vi "MicrophoneColdSpray_Complete_Descriptors_v10.vi"() -> ()   [LabVIEW 2015]
uses:
  <vilib>/Analysis/4window.llb/Hanning Window (DBL).vi
  <vilib>/Analysis/4window.llb/Hamming Window (DBL).vi
  <vilib>/Analysis/4window.llb/Blackman-Harris Window (DBL).vi
  <vilib>/Analysis/4window.llb/Exact Blackman Window (DBL).vi
  <vilib>/Analysis/4window.llb/Blackman Window (DBL).vi
  <vilib>/Analysis/4window.llb/Flat Top Window (DBL).vi
  <vilib>/Analysis/4window.llb/Blackman-Nuttall Window (DBL).vi
  <vilib>/Analysis/4window.llb/Triangle Window (DBL).vi
  <vilib>/Analysis/4window.llb/Modified Bartlett-Hanning Window (DBL).vi
  <vilib>/Analysis/4window.llb/Bohman Window (DBL).vi
  <vilib>/Analysis/4window.llb/Parzen Window (DBL).vi
  <vilib>/Analysis/4window.llb/Welch Window (DBL).vi
  <vilib>/Analysis/4window.llb/AllCosWindow (DBL).vi
  <vilib>/Analysis/0measdsp.llb/Scaled Time Domain Window (DBL).vi
  <vilib>/Analysis/NI_AALPro.lvlib
panel:
  in  "Window Type":u16(ring) items=["Rectangle", "Hanning", "Hamming", "Blackman-Harris", "Exact Blackman", "Blackman", "Flat Top", "Empty1", "Empty2", "Empty3", "Empty4", "Blackman Nuttall", "Empty5", "Empty6", "Empty7", "Empty8", "Empty9", "Empty10", "Empty11", "Empty12", "Empty13", "Empty14", "Empty15", "Empty16", "Empty17", "Empty18", "Empty19", "Empty20", "Empty21", "Empty22", "Triangle", "Bartlett-Hanning", "Bohman", "Parzen", "Welch"]
  out "Boolean 3":bool=TRUE
  out "Boolean 2":bool=TRUE
  out "Boolean":bool=TRUE
  out "DPC":string
  out "Queue Status Check":string
  out "DAC":string
  out "Number of Elements in Queue":i32(knob) scale=0.0..15.0
  out "Microphone Sensitivity":i32=450
  in  "Path to Save Folder for Collected Sound Data":path=path "H:/LabVIEW 2015 Projects/ColdSprayMic/TestDev"
  out "Signal 1":bool
  out "Signal 3":bool
  out "Signal 2":bool
  in  "Noise Amplitude (V) 3":dbl=0.01
  in  "Amplitude (V) 3":dbl=0.3
  in  "Frequency (Hz) 3":dbl=5000.0
  in  "Noise Amplitude (V) 2":dbl=0.02
  in  "Amplitude (V) 2":dbl=0.5
  in  "Frequency (Hz) 2":dbl=2000.0
  in  "Noise Amplitude (V)":dbl=0.3
  in  "Amplitude (V)":dbl=1.0
  in  "Frequency (Hz)":dbl=500.0
  in  "Real Data?":u16(ring) items=["Yes", "No"]
  out "Baseline Spectral Centroid":dbl
  out "Baseline Spectral Spread":dbl
  out "Spectal Descriptors":cluster{dbl, dbl, "t":dbl, dbl}(graph)
  out "Rolling STFT":dbl[][](graph)
  in  "Device Name":tag="cDAQ1Mod1"
  in  "Rate (Hz)":dbl=51200.0
  in  "Number of Samples per Read":i32=4096
  in  "Rolling Buffer (s) MAX 20s":dbl=4.0
  out "Start Time and Date":timestamp
  in  "File Name for Collected Sound Data":string="TestName"
  out "Live Audio":dynamicdata(graph) caption="Waveform Chart"
  in  "stop (F)":bool caption="Stop"
  # "Settings"
  # "Live Signal and Processing"
  # "Real Data = Yes"
  # "Real Data = No"
  # "Simulated Signals"
  # "- Settings for Simulated Signal\n- 10 secs of Signal 1, 10s of Signal 1+2, 10s of Signal 1+2+3, 10s of Signal 1+2, and repeat\n- Set \"Number of Samples per Read\" to 4096 to test with Simulated Signals"
  # "Simulated Signal 1 - Baseline - Sine with Inverse F Noise"
  # "Current Signals"
  # "Program Status"
  # "Simulated Signal 2 - Sine with Inverse F Noise"
  # "Simulated Signal 3  - Sine with Inverse F Noise"
  # "For All Testing"
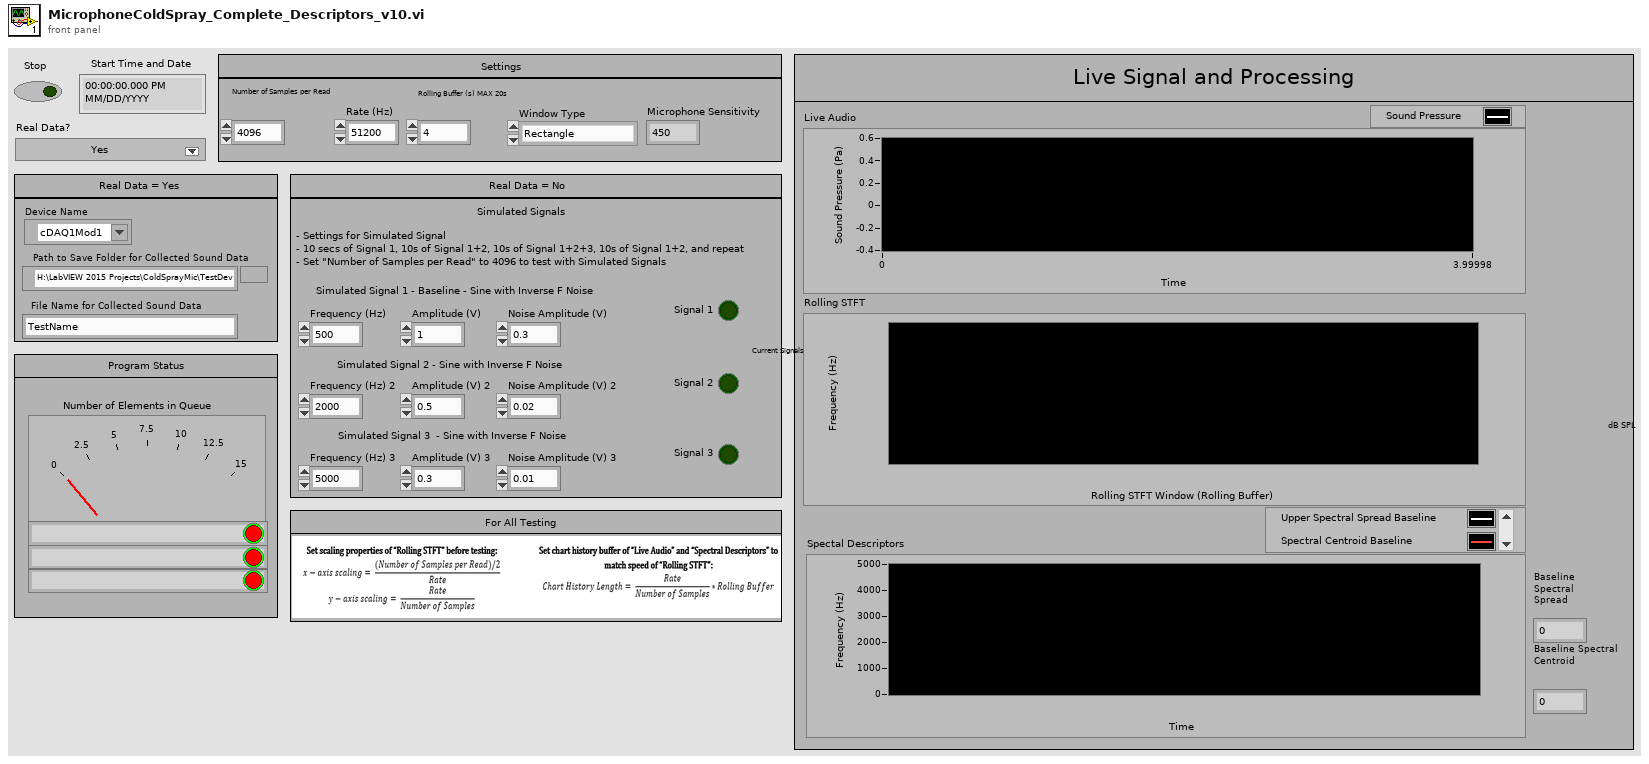
[diagram p1: front panel]
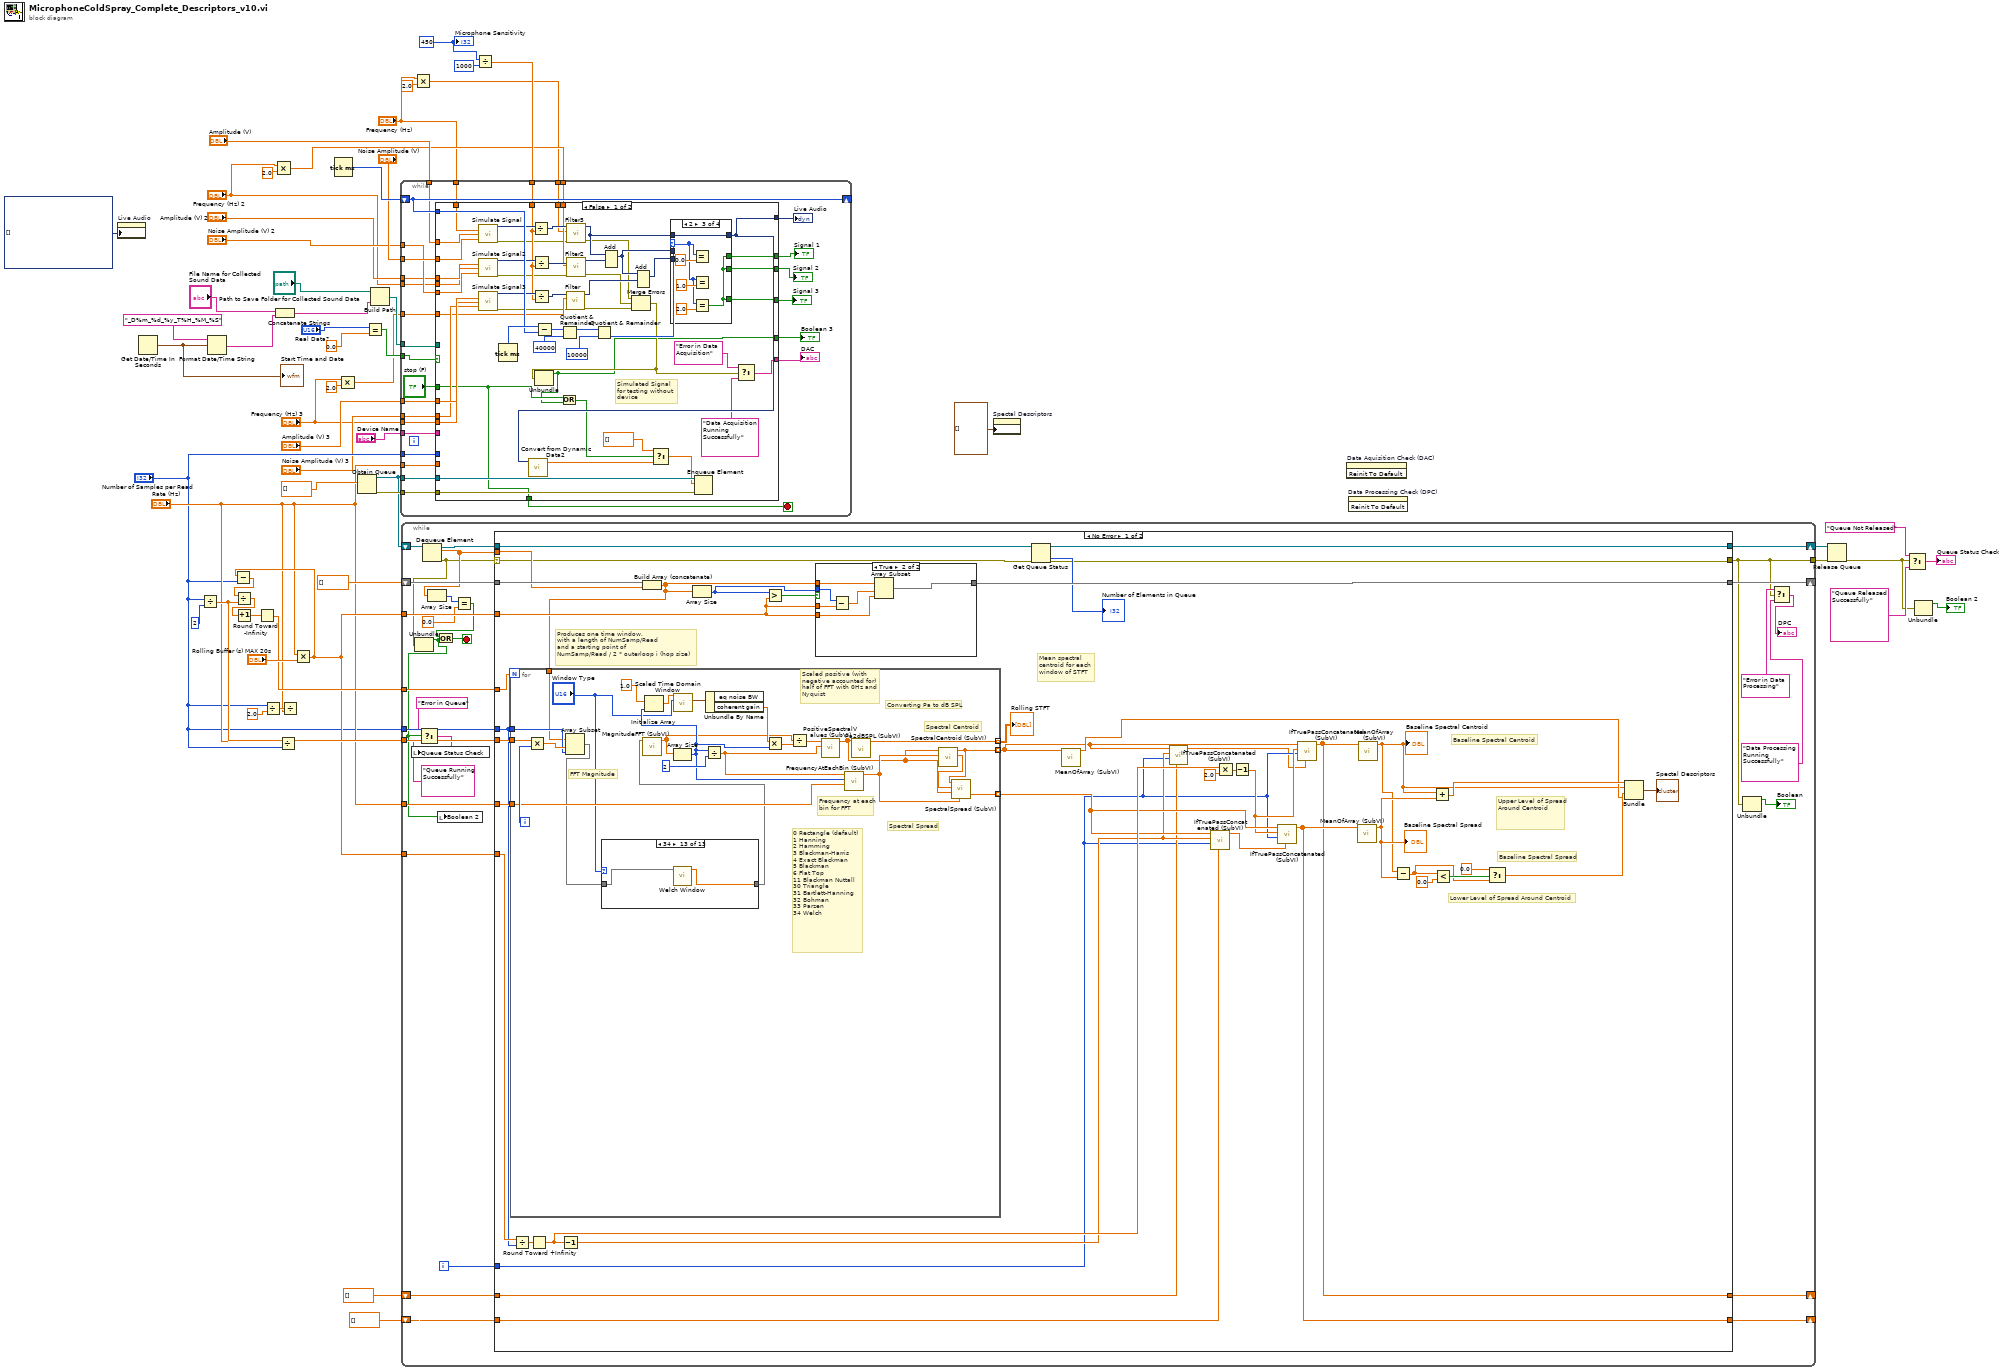
[diagram p0: block diagram]
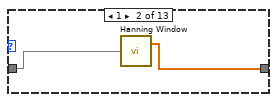
[diagram p4: hidden frame]
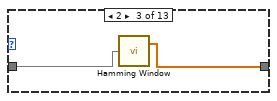
[diagram p5: hidden frame]
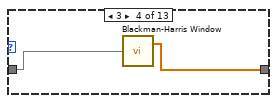
[diagram p6: hidden frame]
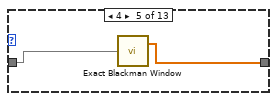
[diagram p7: hidden frame]
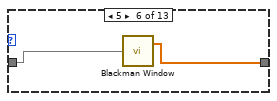
[diagram p8: hidden frame]
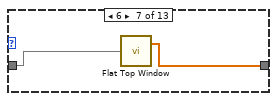
[diagram p9: hidden frame]
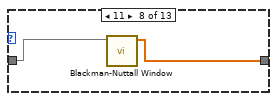
[diagram p10: hidden frame]
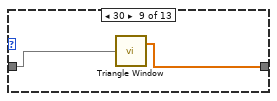
[diagram p11: hidden frame]
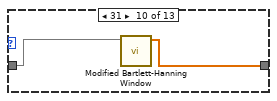
[diagram p12: hidden frame]
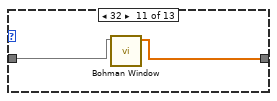
[diagram p13: hidden frame]
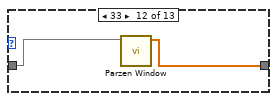
[diagram p14: hidden frame]
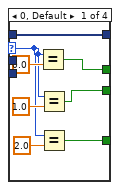
[diagram p16: hidden frame]
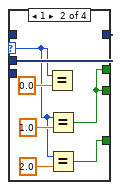
[diagram p17: hidden frame]
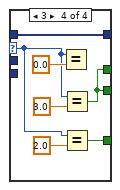
[diagram p18: hidden frame]
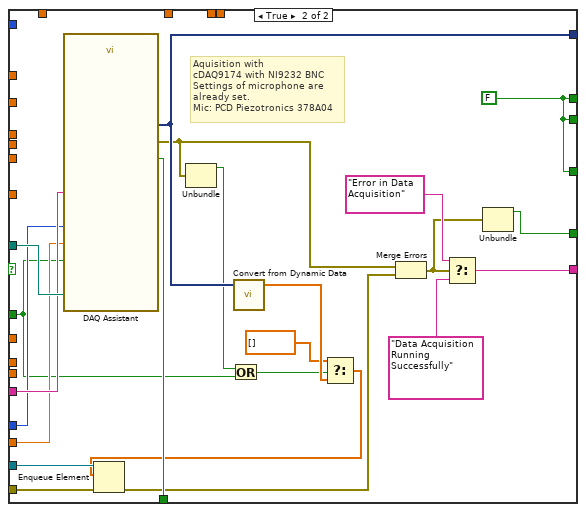
[diagram p19: hidden frame]
diagram:
  w22 = 450
  n1 = property on="Live Audio" class="WFChart (strict)"("History Data"=dynamicdata[] []) -> ()  [unwired: 2 in, 2 out]
  n2 = Get Date/Time In Seconds() -> (seconds since 1Jan1904=w53:timestamp)
  "Start Time and Date" <- w53
  n3 = Divide(x="Number of Samples per Read", y=2) -> (x/y=w45:dbl)
  n4 = Format Date/Time String(time format string (%c)="_D%m_%d_%y_T%H_%M_%S", seconds (now)=w53) -> (date/time string=w55:string)  [unwired: 1 in]
  n5 = Divide(x="Number of Samples per Read", y=2.0) -> (x/y=w38:dbl)
  n6 = Multiply(x="Frequency (Hz) 2", y=2.0) -> (x*y=w15:dbl)
  n7 = Concatenate Strings("File Name for Collected Sound Data", w55) -> (w54:string)
  n8 = Divide(x="Rate (Hz)", y="Number of Samples per Read") -> ()  [unwired: 1 out]
  n9 = Divide(x=w38, y="Rate (Hz)") -> ()  [unwired: 1 out]
  n10 = Multiply(x="Rate (Hz)", y="Rolling Buffer (s) MAX 20s") -> (x*y=w40:dbl)
  n11 = Subtract(x=w40, y="Number of Samples per Read") -> (x-y=w47:dbl)
  n12 = Divide(x=w47, y=w45) -> (x/y=w50:dbl)
  n13 = Increment(x=w50) -> (x+1=w49:dbl)
  n14 = Round Toward -Infinity(1:w49) -> (0:w44:dbl)
  n15 = Tick Count (ms)() -> (millisecond timer value=w31:u32)
  n16 = Multiply(x="Frequency (Hz) 3", y=2.0) -> (x*y=w19:dbl)
  n17 = Obtain Queue(element data type=dbl[] []) -> (queue out=w9:refnum<queue>, error out=w10:errorcluster)  [unwired: 4 in, 1 out]
  n18 = Equal?(x="Real Data?", y=0.0) -> (x = y?=w32:bool)
  n19 = Build Path(base path="Path to Save Folder for Collected Sound Data", name or relative path=w54) -> (appended path=w52:path)
  n20 = while {
    tunnel: w45 -> [w88]
    tunnel: w44 -> [w87]
    tunnel: "Number of Samples per Read" -> [w75]
    tunnel: w40 -> [w86]
    shift-right: [w82] -> _
    shift-left: dbl[] [] -> [w85]
    shift-right: [w83] -> _
    shift-left: dbl[] [] -> [w84]
    tunnel: w40 -> [w81]
    shift-right: [w80] -> w7
    shift-left: w9 -> [w74]
    shift-right: [w79] -> _
    shift-left: dbl[] [] -> [w76]
    tunnel: "Rate (Hz)" -> [w78]
    tunnel: [w59] -> w6
    i -> [w77]
    stop <- w71 stop-if-true
    n21 = Dequeue Element(queue=w74) -> (queue out=w73:refnum<queue>, element=w68:dbl[], error out=w61:errorcluster)  [unwired: 2 in, 1 out]
    n22 = Unbundle(w61) -> ("status"=w58:bool)  [unwired: 2 out]
    n23 = Select(t="Error in Queue", s=w58, f="Queue Running Successfully") -> (s? t:f=w62:string)
    n24 = local write "Queue Status Check"(w62) -> ()
    n25 = Array Size(array=w68) -> (size(s)=w69:i32)
    n26 = local write "Boolean 2"(w58) -> ()
    n27 = Equal?(x=w69, y=0.0) -> (x = y?=w72:bool)
    n28 = Or(x=w72, y=w58) -> (x .or. y?=w71:bool)
    n29 = case shown="No Error" w61 {
      selector: w61 -> [w89 w189]
      tunnel: w88 -> [w118 _]
      tunnel: w87 -> [w117 _]
      tunnel: w86 -> [w116 _]
      tunnel: w85 -> [w99 w193]
      tunnel: w84 -> [w115 w192]
      tunnel: [w103 w192] -> w83
      tunnel: [w94 w193] -> w82
      tunnel: w81 -> [w112 _]
      tunnel: [w92 w190] -> w80
      tunnel: [w111 w191] -> w79
      tunnel: w78 -> [w110 _]
      tunnel: w77 -> [w97 _]
      tunnel: w76 -> [w108 w191]
      tunnel: w75 -> [w107 _]
      tunnel: w73 -> [w93 w190]
      tunnel: w68 -> [w106 _]
      tunnel: [w90 w189] -> w59
      frame No Error {
        # "Produces one time window,\nwith a length of NumSamp/Read\nand a starting point of \nNumSamp/Read / 2 * outerloop i (hop size)"
        # "Mean spectral centroid for each window of STFT"
        # "Upper Level of Spread Around Centroid"
        # "Lower Level of Spread Around Centroid"
        # "Baseline Spectral Centroid"
        # "Baseline Spectral Spread"
        n30 = Divide(x=w116, y=w107) -> (x/y=w130:dbl)
        n31 = Round Toward +Infinity(x=w130) -> (ceil(x): smallest int >= x=w127:dbl)
        n32 = Decrement(x=w127) -> (x-1=w100:dbl)
        n33 = Build Array (concatenate)(w108, w106) -> (w109:dbl[])
        n34 = for {
          N: w117 -> [_]
          tunnel: [w161] -> w131 mode=indexing
          tunnel: [w159] -> w96 mode=indexing
          tunnel: [w156] -> w104 mode=indexing
          tunnel: w118 -> [w154]
          tunnel: w107 -> [w153]
          tunnel: w110 -> [w152]
          tunnel: w109 -> [w151]
          i -> [w160]
          # "0 Rectangle (default) \n1 Hanning \n2 Hamming \n3 Blackman-Harris \n4 Exact Blackman \n5 Blackman \n6 Flat Top \n11 Blackman Nuttall \n30 Triangle \n31 Bartlett-Hanning \n32 Bohman \n33 Parzen \n34 Welch"
          # "FFT Magnitude"
          # "Converting Pa to dB SPL"
          # "Scaled positive (with negative accounted for) half of FFT with 0Hz and Nyquist"
          # "Frequency at each bin for FFT"
          # "Spectral Spread"
          # "Spectral Centroid"
          n35 = Multiply(x=w154, y=w160) -> (x*y=w163:dbl)
          n36 = Array Subset(array=w151, index=w163, length=w153) -> (w141:dbl[])
          n37 = case shown="34" "Window Type" {
            tunnel: w141 -> [w164 w166 w168 w170 w172 w174 w176 w178 w180 w182 w184 w186 w188]
            tunnel: [w164 w165 w167 w169 w171 w173 w175 w177 w179 w181 w183 w185 w187] -> w140
            frame 0, Default {
            }
            frame 1 {
              n38 = call-poly <vilib>:"Hanning Window.vi"("X"=w166) -> ("Windowed X"=w165:dbl[])  [unwired: 1 out]
            }
            frame 2 {
              n39 = call-poly <vilib>:"Hamming Window.vi"("X"=w168) -> ("Windowed X"=w167:dbl[])  [unwired: 1 out]
            }
            frame 3 {
              n40 = call-poly <vilib>:"Blackman-Harris Window.vi"("X"=w170) -> ("Windowed X"=w169:dbl[])  [unwired: 1 out]
            }
            frame 4 {
              n41 = call-poly <vilib>:"Exact Blackman Window.vi"("X"=w172) -> ("Windowed X"=w171:dbl[])  [unwired: 1 out]
            }
            frame 5 {
              n42 = call-poly <vilib>:"Blackman Window.vi"("X"=w174) -> ("Windowed X"=w173:dbl[])  [unwired: 1 out]
            }
            frame 6 {
              n43 = call-poly <vilib>:"Flat Top Window.vi"("X"=w176) -> ("Windowed X"=w175:dbl[])  [unwired: 1 out]
            }
            frame 11 {
              n44 = call-poly <vilib>:"Blackman-Nuttall Window.vi"("X"=w178) -> ("Windowed X"=w177:dbl[])  [unwired: 9 in, 1 out]
            }
            frame 30 {
              n45 = call-poly <vilib>:"Triangle Window.vi"("X"=w180) -> ("Windowed X"=w179:dbl[])  [unwired: 1 out]
            }
            frame 31 {
              n46 = call-poly <vilib>:"Modified Bartlett-Hanning Window.vi"("X"=w182) -> ("Windowed X"=w181:dbl[])  [unwired: 9 in, 1 out]
            }
            frame 32 {
              n47 = call-poly <vilib>:"Bohman Window.vi"("X"=w184) -> ("Windowed X"=w183:dbl[])  [unwired: 9 in, 1 out]
            }
            frame 33 {
              n48 = call-poly <vilib>:"Parzen Window.vi"("X"=w186) -> ("Windowed X"=w185:dbl[])  [unwired: 9 in, 1 out]
            }
            frame 34 {
              n49 = call-poly <vilib>:"Welch Window.vi"("X"=w188) -> ("Windowed X"=w187:dbl[])  [unwired: 9 in, 1 out]
            }
          }
          n50 = call "MagnitudeFFT (SubVI).vi"("Windowed Signal Array"=w140) -> ("Magnitude FFT"=w143:dbl[])  [unwired: 10 in]
          n51 = Array Size(array=w143) -> (size(s)=w144:i32)
          n52 = Initialize Array(1.0 ("element"), w144) -> (w145:dbl[])
          n53 = call-poly <vilib>:"Scaled Time Domain Window.vi"("window"="Window Type", "X"=w145) -> ("window properties"=w148:cluster{"eq noise BW":dbl, "coherent gain":dbl})  [unwired: 1 in, 8 out]
          n54 = Unbundle By Name(w148) -> ("coherent gain"=w147:dbl)  [unwired: 1 out]
          n55 = Divide(x=w144, y=2) -> (x/y=w155:dbl)
          n56 = Multiply(x=w147, y=w144) -> (x*y=w146:dbl)
          n57 = Divide(x=w143, y=w146) -> (x/y=w142:dbl[])
          n58 = call "PositiveSpectralValues (SubVI).vi"("Size of Positive Half of FFT"=w155, "Scaled Full Length FFT"=w142) -> ("Positve Half of FFT with 0Hz and Nyquist"=w150:dbl[])  [unwired: 9 in]
          n59 = call "FrequencyAtEachBin (SubVI).vi"("Rate of Measurement (Hz)"=w152, "Length of Full FFT"=w144, "Length of Positive Half of FFT"=w155) -> ("Frequency Array"=w158:dbl[])  [unwired: 8 in]
          n60 = call "Pa2dBSPL (SubVI).vi"("Positve Half of FFT with 0Hz and Nyquist"=w150) -> ("dB SPL"=w161:dbl[])  [unwired: 10 in]
          n61 = call "SpectralCentroid (SubVI).vi"("Frequency Array"=w158, "Positve Half of FFT with 0Hz and Nyquist"=w150) -> ("Sum of FFT Mags"=w157:dbl, "Spectral Centroid"=w159:dbl)  [unwired: 8 in]
          n62 = call "SpectralSpread (SubVI).vi"("Frequency Array"=w158, "Positve Half of FFT with 0Hz and Nyquist"=w150, "Sum of FFT Mags"=w157, "Spectral Centroid"=w159) -> ("Spectral Spread"=w156:dbl)  [unwired: 7 in]
        }
        "Rolling STFT" <- w131
        n63 = Array Size(array=w109) -> (size(s)=w114:i32)
        n64 = Greater?(x=w114, y=w112) -> (0:w113:bool)
        n65 = case shown="True" w113 {
          tunnel: w109 -> [w132 w138]
          tunnel: w112 -> [_ w137]
          tunnel: w114 -> [_ w135]
          tunnel: w112 -> [_ w134]
          tunnel: [w132 w133] -> w111
          frame False {
          }
          frame True {
            n66 = Subtract(x=w135, y=w134) -> (x-y=w136:dbl)
            n67 = Array Subset(array=w138, index=w136, length=w137) -> (w133:dbl[])
          }
        }
        n68 = Get Queue Status(queue=w93, error in (no error)=w89) -> (queue out=w92:refnum<queue>, error out=w90:errorcluster, # elements in queue=→"Number of Elements in Queue":i32)  [unwired: 1 in, 5 out]
        n69 = call "MeanOfArray (SubVI).vi"("Array"=w96) -> ("Mean"=w120:dbl)  [unwired: 10 in]
        n70 = call "IfTruePassConcatenated (SubVI).vi"("Old Array"=w99, "Loop Number"=w97, "Condition"=w100, "New Array"=w96) -> ("If True, Concatenated"=w95:dbl[])  [unwired: 7 in]
        n71 = call "IfTruePassConcatenated (SubVI).vi"("Old Array"=w115, "Loop Number"=w97, "Condition"=w100, "New Array"=w104) -> ("If True, Concatenated"=w105:dbl[])  [unwired: 7 in]
        n72 = Multiply(x=w127, y=2.0) -> (x*y=w128:dbl)
        n73 = Decrement(x=w128) -> (x-1=w98:dbl)
        n74 = call "IfTruePassConcatenated (SubVI).vi"("Old Array"=w105, "Loop Number"=w97, "Condition"=w98, "New Array"=w104) -> ("If True, Concatenated"=w103:dbl[])  [unwired: 7 in]
        n75 = call "IfTruePassConcatenated (SubVI).vi"("Old Array"=w95, "Loop Number"=w97, "Condition"=w98, "New Array"=w96) -> ("If True, Concatenated"=w94:dbl[])  [unwired: 7 in]
        n76 = call "MeanOfArray (SubVI).vi"("Array"=w103) -> ("Mean"=w102:dbl)  [unwired: 10 in]
        "Baseline Spectral Spread" <- w102
        n77 = call "MeanOfArray (SubVI).vi"("Array"=w94) -> ("Mean"=w101:dbl)  [unwired: 10 in]
        "Baseline Spectral Centroid" <- w101
        n78 = Subtract(x=w101, y=w102) -> (x-y=w123:dbl)
        n79 = Add(x=w101, y=w102) -> (x+y=w122:dbl)
        n80 = Less?(x=w123, y=0.0) -> (x < y?=w125:bool)
        n81 = Select(t=0.0, s=w125, f=w123) -> (s? t:f=w121:dbl)
        n82 = Bundle(w122, "Mean"=w101, "t"=w121, "Mean"=w120) -> (→"Spectal Descriptors":cluster{dbl, "Mean":dbl, "t":dbl, "Mean":dbl})  [unwired: 1 in]
      }
      frame Error {
      }
    }
    n83 = Unbundle(w59) -> ("status"=→"Boolean":bool)  [unwired: 2 out]
    n84 = Select(t="Error in Data Processing", s=w59, f="Data Processing Running Successfully") -> (s? t:f=→"DPC":string)
  }
  n85 = Multiply(x="Frequency (Hz)", y=2.0) -> (x*y=w13:dbl)
  n86 = Divide(x=w22, y=1000) -> (x/y=w21:dbl)
  n87 = while {
    tunnel: w52 -> [w221]
    tunnel: "Device Name" -> [w220]
    tunnel: "Rate (Hz)" -> [w219]
    tunnel: "Number of Samples per Read" -> [w218]
    tunnel: w32 -> [w215]
    shift-right: [w214] -> _
    shift-left: w31 -> [w214]
    tunnel: "Frequency (Hz)" -> [w213]
    tunnel: "Amplitude (V)" -> [w212]
    tunnel: "Noise Amplitude (V)" -> [w211]
    tunnel: "Noise Amplitude (V) 2" -> [w210]
    tunnel: "Amplitude (V) 2" -> [w209]
    tunnel: "Frequency (Hz) 2" -> [w208]
    tunnel: "Frequency (Hz) 3" -> [w207]
    tunnel: "Amplitude (V) 3" -> [w206]
    tunnel: "Noise Amplitude (V) 3" -> [w205]
    tunnel: w21 -> [w204]
    tunnel: w19 -> [w203]
    tunnel: w15 -> [w202]
    tunnel: w13 -> [w201]
    tunnel: w9 -> [w197]
    tunnel: w10 -> [w196]
    stop <- w217 stop-if-true
    n88 = case shown="False" w215 {
      tunnel: "stop (F)" -> [w229 w312]
      tunnel: w221 -> [_ w325]
      tunnel: w220 -> [_ w324]
      tunnel: w219 -> [_ w323]
      tunnel: w218 -> [_ w322]
      tunnel: w196 -> [w275 w321]
      tunnel: [w229 w320] -> w217
      tunnel: [w266 w319] -> w216
      tunnel: w214 -> [w273 _]
      tunnel: w213 -> [w265 _]
      tunnel: w212 -> [w264 _]
      tunnel: w211 -> [w263 _]
      tunnel: w210 -> [w262 _]
      tunnel: w209 -> [w261 _]
      tunnel: w208 -> [w260 _]
      tunnel: w207 -> [w259 _]
      tunnel: w206 -> [w258 _]
      tunnel: w205 -> [w257 _]
      tunnel: w204 -> [w246 _]
      tunnel: w203 -> [w245 _]
      tunnel: w202 -> [w244 _]
      tunnel: w201 -> [w243 _]
      tunnel: [w242 w318] -> w200
      tunnel: [w241 w318] -> w199
      tunnel: [w240 w318] -> w198
      tunnel: w197 -> [w239 w317]
      tunnel: [w225 w306] -> w195
      tunnel: [w223 w304] -> w194
      frame False {
        # "Simulated Signal\nfor testing without\ndevice"
        n89 = call "Simulate Signal"("Frequency"=w265, "Amplitude"=w264, "Noise amplitude"=w263) -> ("Sine with Inverse F Noise"=w251:dynamicdata, "error out"=w233:errorcluster)  [unwired: 11 in]
        n90 = call "Simulate Signal2"("Frequency"=w260, "Amplitude"=w261, "Noise amplitude"=w262) -> ("Sine with Inverse F Noise"=w250:dynamicdata, "error out"=w234:errorcluster)  [unwired: 11 in]
        n91 = call "Simulate Signal3"("Frequency"=w259, "Amplitude"=w258, "Noise amplitude"=w257) -> ("Sine with Inverse F Noise"=w247:dynamicdata, "error out"=w235:errorcluster)  [unwired: 11 in]
        n92 = Tick Count (ms)() -> (millisecond timer value=w274:u32)
        n93 = Divide(x=w251, y=w246) -> (x/y=w252:dynamicdata)
        n94 = Divide(x=w250, y=w246) -> (x/y=w249:dynamicdata)
        n95 = Divide(x=w247, y=w246) -> (x/y=w248:dynamicdata)
        n96 = Subtract(x=w274, y=w273) -> (x-y=w272:u32)
        n97 = Quotient & Remainder(x=w272, y=u32 40000) -> (x-y*floor(x/y)=w270:u32)  [unwired: 1 out]
        n98 = call "Filter"("error in (no error)"=w235, "Upper Cut-Off"=w245, "Signal"=w248) -> ("error out"=w230:errorcluster, "Filtered Signal"=w254:dynamicdata)  [unwired: 7 in]
        n99 = call "Filter3"("error in (no error)"=w233, "Upper Cut-Off"=w243, "Signal"=w252) -> ("error out"=w232:errorcluster, "Filtered Signal"=w253:dynamicdata)  [unwired: 7 in]
        n100 = call "Filter2"("error in (no error)"=w234, "Upper Cut-Off"=w244, "Signal"=w249) -> ("error out"=w231:errorcluster, "Filtered Signal"=w255:dynamicdata)  [unwired: 7 in]
        n101 = Quotient & Remainder(x=w270, y=u32 10000) -> (floor(x/y)=w256:u32)  [unwired: 1 out]
        n102 = Add(1:w255, 2:w253) -> (0:w268:dynamicdata)  [unwired: 1 in, 1 out]
        n103 = Merge Errors(w232, w231, w230) -> (w224:errorcluster)
        n104 = Unbundle(w224) -> ("status"=w223:bool)  [unwired: 2 out]
        n105 = Or(x=w229, y=w223) -> (x .or. y?=w228:bool)
        n106 = Add(1:w254, 2:w268) -> (0:w267:dynamicdata)  [unwired: 1 in, 1 out]
        n107 = case shown="2" w256 {
          selector: w256 -> [w277 w284 w291 w300]
          tunnel: w253 -> [w283 _ _ _]
          tunnel: [w283 w290 w296 w298] -> w266
          tunnel: w268 -> [_ w290 _ w298]
          tunnel: w267 -> [_ _ w296 _]
          tunnel: [w279 w286 w292 w297] -> w242
          tunnel: [w276 w286 w292 w297] -> w241
          tunnel: [w278 w285 w292 w299] -> w240
          frame 0, Default {
            n108 = Equal?(x=w277, y=0.0) -> (x = y?=w279:bool)
            n109 = Equal?(x=w277, y=1.0) -> (x = y?=w276:bool)
            n110 = Equal?(x=w277, y=2.0) -> (x = y?=w278:bool)
          }
          frame 1 {
            n111 = Equal?(x=w284, y=0.0) -> ()  [unwired: 1 out]
            n112 = Equal?(x=w284, y=1.0) -> (x = y?=w286:bool)
            n113 = Equal?(x=w284, y=2.0) -> (x = y?=w285:bool)
          }
          frame 2 {
            n114 = Equal?(x=w291, y=0.0) -> ()  [unwired: 1 out]
            n115 = Equal?(x=w291, y=1.0) -> ()  [unwired: 1 out]
            n116 = Equal?(x=w291, y=2.0) -> (x = y?=w292:bool)
          }
          frame 3 {
            n117 = Equal?(x=w300, y=0.0) -> ()  [unwired: 1 out]
            n118 = Equal?(x=w300, y=3.0) -> (x = y?=w297:bool)
            n119 = Equal?(x=w300, y=2.0) -> (x = y?=w299:bool)
          }
        }
        n120 = call "Convert from Dynamic Data2"("Dynamic Data Type"=w266) -> ("Array"=w237:dbl[])  [unwired: 3 in]
        n121 = Select(t=dbl[] [], s=w228, f=w237) -> (s? t:f=w236:dbl[])
        n122 = Enqueue Element(queue=w239, element=w236, error in (no error)=w275) -> ()  [unwired: 1 in, 3 out]
        n123 = Select(t="Error in Data Acquisition", s=w224, f="Data Acquisition Running Successfully") -> (s? t:f=w225:string)
      }
      frame True {
        w318 = FALSE
        # "Aquisition with\ncDAQ9174 with NI9232 BNC\nSettings of microphone are \nalready set. \nMic: PCD Piezotronics 378A04"
        n124 = call "DAQ Assistant"("rate"=w323, "number of samples"=w322, "stop (F)"=w312, "file path"=w325, "device name"=w324) -> ("data"=w319:dynamicdata, "stopped"=w320:bool, "error out"=w309:errorcluster)  [unwired: 11 in, 1 out]
        n125 = Unbundle(w309) -> ("status"=w313:bool)  [unwired: 2 out]
        n126 = Or(x=w313, y=w312) -> (x .or. y?=w311:bool)
        n127 = call "Convert from Dynamic Data"("Dynamic Data Type"=w319) -> ("Array"=w316:dbl[])  [unwired: 3 in]
        n128 = Select(t=dbl[] [], s=w311, f=w316) -> (s? t:f=w314:dbl[])
        n129 = Enqueue Element(queue=w317, element=w314, error in (no error)=w321) -> (error out=w310:errorcluster)  [unwired: 1 in, 2 out]
        n130 = Merge Errors(w309, w310) -> (w305:errorcluster)
        n131 = Select(t="Error in Data Acquisition", s=w305, f="Data Acquisition Running Successfully") -> (s? t:f=w306:string)
        n132 = Unbundle(w305) -> ("status"=w304:bool)  [unwired: 2 out]
      }
    }
    "Live Audio" <- w216
    "Signal 1" <- w200
    "Signal 2" <- w199
    "Signal 3" <- w198
    "DAC" <- w195
    "Boolean 3" <- w194
  }
  n133 = property on="Spectal Descriptors" class="WFChart (strict)"("History Data"=cluster{dbl, dbl, "t":dbl, dbl}[] []) -> ()  [unwired: 2 in, 2 out]
  n134 = invoke on="Data Aquisition Check (DAC)" class="Str" method="Reinit To Default"() -> ()  [unwired: 3 in, 3 out]
  n135 = invoke on="Data Processing Check (DPC)" class="Str" method="Reinit To Default"() -> ()  [unwired: 3 in, 3 out]
  n136 = Release Queue(queue=w7, error in (no error)=w6) -> (error out=w2:errorcluster)  [unwired: 1 in, 2 out]
  n137 = Select(t="Queue Not Released", s=w2, f="Queue Released Successfully" ("t")) -> (s? t:f=→"Queue Status Check":string)
  n138 = Unbundle(w2) -> ("status"=→"Boolean 2":bool)  [unwired: 2 out]
  "Microphone Sensitivity" <- w22
